vi "TDTRX6-Start.vi"(4 "error in (no error)":errorcluster) -> (0 "error out":errorcluster)   [LabVIEW 2015]
doc: "Sends <B>Start</B> notifier to DAQ thread to begin measurement."
uses:
  TDT-Globals.vi
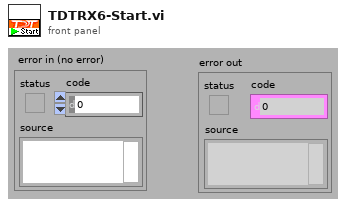
[diagram p1: front panel]
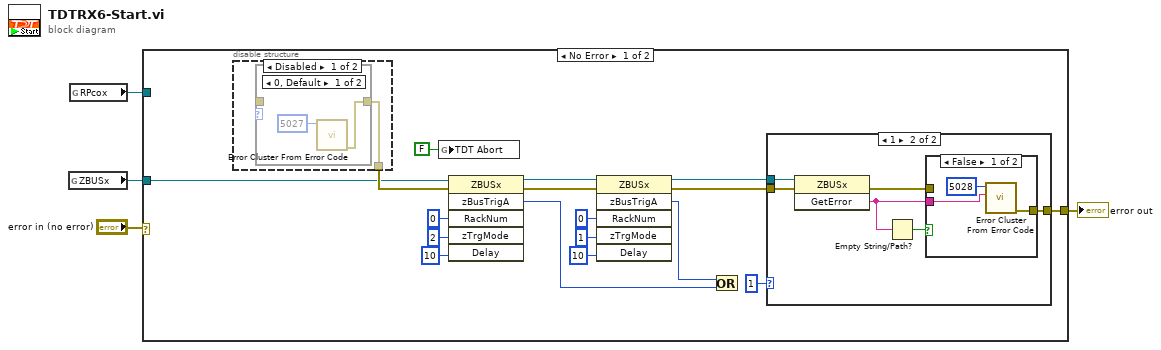
[diagram p0: block diagram]
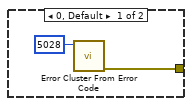
[diagram p4: hidden frame]
diagram:
  n1 = global read "TDT-Globals.vi" "ZBUSx"() -> (w3:refnum<k7>)
  n2 = global read "TDT-Globals.vi" "RPcox"() -> (w1:refnum<k7>)
  n3 = case shown="No Error" "error in (no error)" {
    selector: "error in (no error)" -> [_ w38]
    tunnel: [w11 w38] -> w2
    tunnel: w3 -> [w5 _]
    tunnel: w1 -> [_ _]
    frame No Error {
      n4 = disable-structure shown="Disabled" {
        disable-tunnel: [w22 _] -> w6
        frame Disabled {
          n5 = case shown="0, Default" {
            selector: _ -> [_ _]
            tunnel: _ -> [_ w25]
            tunnel: [w23 w25] -> w22
            frame 0, Default {
              n6 = call <vilib>:"Error Cluster From Error Code.vi"("error code (0)"=5027) -> ("error out"=w23:errorcluster)  [unwired: 8 in]
            }
            frame 1 {
            }
          }
        }
        frame Enabled {
        }
      }
      n7 = global write "TDT-Globals.vi" "TDT Abort"(FALSE ("TDT Abort")) -> ()
      n8 = invoke class="ZBUSx" method="zBusTrigA"(reference=w5, error in=w6, "RackNum"=0, "zTrgMode"=2, "Delay"=10) -> (reference out=w15:refnum<k7>, error out=w14:errorcluster, "zBusTrigA"=w12:i32)  [unwired: 1 in, 3 out]
      n9 = invoke class="ZBUSx" method="zBusTrigA"(reference=w15, error in=w14, "RackNum"=0, "zTrgMode"=1, "Delay"=10) -> (reference out=w9:refnum<k7>, error out=w10:errorcluster, "zBusTrigA"=w13:i32)  [unwired: 1 in, 3 out]
      n10 = Or(x=w13, y=w12) -> ()  [unwired: 1 out]
      n11 = case shown="1" 1 {
        tunnel: [w26 w28] -> w11
        tunnel: w10 -> [_ w33]
        tunnel: w9 -> [_ w32]
        frame 0, Default {
          n12 = call <vilib>:"Error Cluster From Error Code.vi"("error code (0)"=5028) -> ("error out"=w26:errorcluster)  [unwired: 8 in]
        }
        frame 1 {
          n13 = invoke class="ZBUSx" method="GetError"(reference=w32, error in=w33) -> (error out=w31:errorcluster, "GetError"=w29:string)  [unwired: 1 in, 1 out]
          n14 = Empty String/Path?(string/path=w29) -> (empty?=w30:bool)
          n15 = case shown="False" w30 {
            tunnel: w31 -> [_ w37]
            tunnel: w29 -> [w35 _]
            tunnel: [w34 w37] -> w28
            frame False {
              n16 = call <vilib>:"Error Cluster From Error Code.vi"("error message (\"\")"=w35, "error code (0)"=5028) -> ("error out"=w34:errorcluster)  [unwired: 7 in]
            }
            frame True {
            }
          }
        }
      }
    }
    frame Error {
    }
  }
  "error out" <- w2
